vi "MagEncoder_cal_v1.vi"() -> ()   [LabVIEW 2014]
uses:
  <vilib>/eio/EIONode/EIONode.xnode
  <vilib>/rvi/eio/common/nirviEmuTemplateMethod_errors.vi
  <vilib>/rvi/Analysis/measure/butterworth/XNode/niFpgaButterworthFilter.xnode
  <vilib>/rvi/DataTransferAndStorage/Container/XNode/niFpgaContainer.xnode
  <vilib>/rvi/FXPMathLib/FxpSinAndCos/XNode/nifxpmath_SinAndCos.xnode
  <vilib>/rvi/FXPMathLib/FxpSinAndCos/simVIs/DllFxpSinAndCosTemp_sub.vi
  <vilib>/rvi/FXPMathLib/FxpSinAndCos/subVIs/nifxpmath_SinAndCos_SimConfig.ctl
  <vilib>/rvi/interface/RandomDataEmulation/nirviRandomDataFpgaMultiElementTemplate.vi
panel:
  in  "Vy (mm/s)":fxp<+/-,30,6>
  out "Dyr_ramp":fxp<+/-,22,7>
  in  "Dyr_stroke":fxp<+/-,32,7>
  out "Dpr_ramp":fxp<+/-,22,7>
  in  "Dpr_stroke":fxp<+/-,32,7>
  in  "Vp (mm/s)":fxp<+/-,30,6>
  out "omega_p (Mavg w. f)":fxp<+/-,36,18>
  in  "scaled coefficients":i32[](array[numeric])=[946630756, 63555534]
  in  "FIFO":i16(ring) items=["Pitch_F+P", "imp ctrl", "Yaw_F+P"]
  out "PID (kHz)":fxp<+/-,20,10>
  in  "Set 6":bool
  in  "Set 5":bool
  in  "Set 4":bool
  in  "Set 3":bool
  in  "Set 2":bool
  in  "Set 1":bool
  out "Dy1_d (T)":fxp<+/-,36,13>
  out "omega_y1 (T)":fxp<+/-,36,13>
  out "Dp1_d (T)":fxp<+/-,36,13>
  out "omega_p1 (T)":fxp<+/-,36,13>
  out "Dy2_d (T)":fxp<+/-,36,13>
  out "Dp2_d (T)":fxp<+/-,36,13>
  out "omega_y2 (T)":fxp<+/-,36,13>
  out "omega_p2 (T)":fxp<+/-,36,13>
  out "mt_omega_y2":u32
  out "mt_omega_p2":u32
  out "rad_y2":fxp<+/-,33,20>
  out "D_y2":fxp<+/-,32,7>
  out "rad_y1":fxp<+/-,33,20>
  out "D_y1":fxp<+/-,32,7>
  out "Encoder Position_y1":i32
  out "Encoder Position_y2":i32
  out "Encoder Position_p2":i32
  out "D_p2":fxp<+/-,32,7>
  out "rad_p2":fxp<+/-,33,20>
  out "D_p1":fxp<+/-,32,7>
  out "rad_p1":fxp<+/-,33,20>
  out "Encoder Position_p1":i32
  in  "Mag. factor_y":fxp<+/-,20,3>
  in  "Mag. encoder_y":bool
  out "omega_y (rad/s)":fxp<+/-,36,13>
  out "Dy_d (mm/s)":fxp<+/-,36,13>
  in  "Vy. Est.":i16(ring) items=["T", "Mavg"]
  out "omega_y (Mavg)":fxp<+/-,36,14>
  out "Dy_d (Mavg)":fxp<+/-,36,14>
  in  "Dy_d_M_avg_Tc (uSec)":i32
  out "Dp_d (Mavg)":fxp<+/-,36,14>
  out "omega_p (Mavg)":fxp<+/-,36,14>
  in  "Dp_d_M_avg_Tc (uSec)":i32
  out "Dp_d (T)":fxp<+/-,36,13>
  out "omega_p (T)":fxp<+/-,36,13>
  in  "Vp. Est.":i16(ring) items=["T", "Mavg"]
  in  "Mag. factor_p":fxp<+/-,20,3>
  in  "Mag. encoder_p":bool
  in  "Belt_out_p":fxp<+/-,7,7>
  in  "Belt_in_p":fxp<+/-,6,6>
  in  "Belt_out_y":fxp<+/-,7,7>
  in  "Belt_in_y":fxp<+/-,6,6>
  in  "mt0_omega_p":u32
  in  "Encoder reset":bool
  out "Dpr_sin":fxp<+/-,22,7>
  in  "Sin offset_p":fxp<+/-,22,7>
  in  "Sin magnitude_p":fxp<+/-,21,6>
  out "Dpr_sin_dd":fxp<+/-,35,20>
  out "Dpr_sin_d":fxp<+/-,33,15>
  out "Sin omega_p":fxp<+/-,34,9>
  in  "Sin wave freq._p (Hz)":fxp<+/-,32,6>
  in  "Dpr_step":fxp<+/-,22,7>
  out "Dpr_for":fxp<+/-,22,7>
  in  "Command_p":i16(ring) items=["Step", "Sine", "Ramp"]
  out "Fp_PID":fxp<+/-,36,16>
  in  "Kp_p":fxp<+/-,32,13>
  out "va_p":fxp<+/-,36,7>
  out "vb_p":fxp<+/-,37,8>
  out "vq_p_F":fxp<+/-,20,5> format="%.57g"
  out "vd_p_F":fxp<+/-,20,5>
  in  "Stop motor_p":bool
  out "Dp_d (mm/s)":fxp<+/-,36,13>
  out "omega_p (rad/s)":fxp<+/-,36,13>
  out "mt_omega_p1":u32
  out "rad_p(NrTheta)":fxp<+/-,33,20>
  out "D_p(mm)":fxp<+/-,32,7>
  out "Encoder Position_p":i32
  in  "Encoder reset_p":bool
  out "Dyr_for":fxp<+/-,22,7>
  in  "Command_y":i16(ring) items=["Step", "Sine", "Ramp"]
  out "vb_y":fxp<+/-,38,8>
  out "va_y":fxp<+/-,38,8>
  out "Dyr_sin_dd":fxp<+/-,35,20>
  out "Dyr_sin_d":fxp<+/-,33,15>
  out "Sin omega_y":fxp<+/-,34,9>
  out "Dyr_sin":fxp<+/-,22,7>
  in  "Sin offset_y":fxp<+/-,22,7>
  in  "Sin magnitude_y":fxp<+/-,21,6>
  out "Time now(s)":fxp<+,52,14>
  in  "Sin wave freq._y (Hz)":fxp<+/-,32,6>
  in  "Dyr_step":fxp<+/-,22,7>
  out "Fy_PID":fxp<+/-,36,16>
  in  "Kp_y":fxp<+/-,32,13>
  out "vq_y_F":fxp<+/-,20,5> format="%.57g"
  out "vd_y_F":fxp<+/-,20,5>
  in  "Stop motor_y":bool
  out "Dy_d (T)":fxp<+/-,36,13>
  out "omega_y (T)":fxp<+/-,36,13>
  in  "mt0_omega_y":u32
  out "mt_omega_y1":u32
  out "rad_y(NrTheta)":fxp<+/-,33,20>
  out "D_y(mm)":fxp<+/-,32,7>
  out "Encoder Position_y":i32
  in  "Encoder reset_y":bool
  in  "Ini coe.":bool
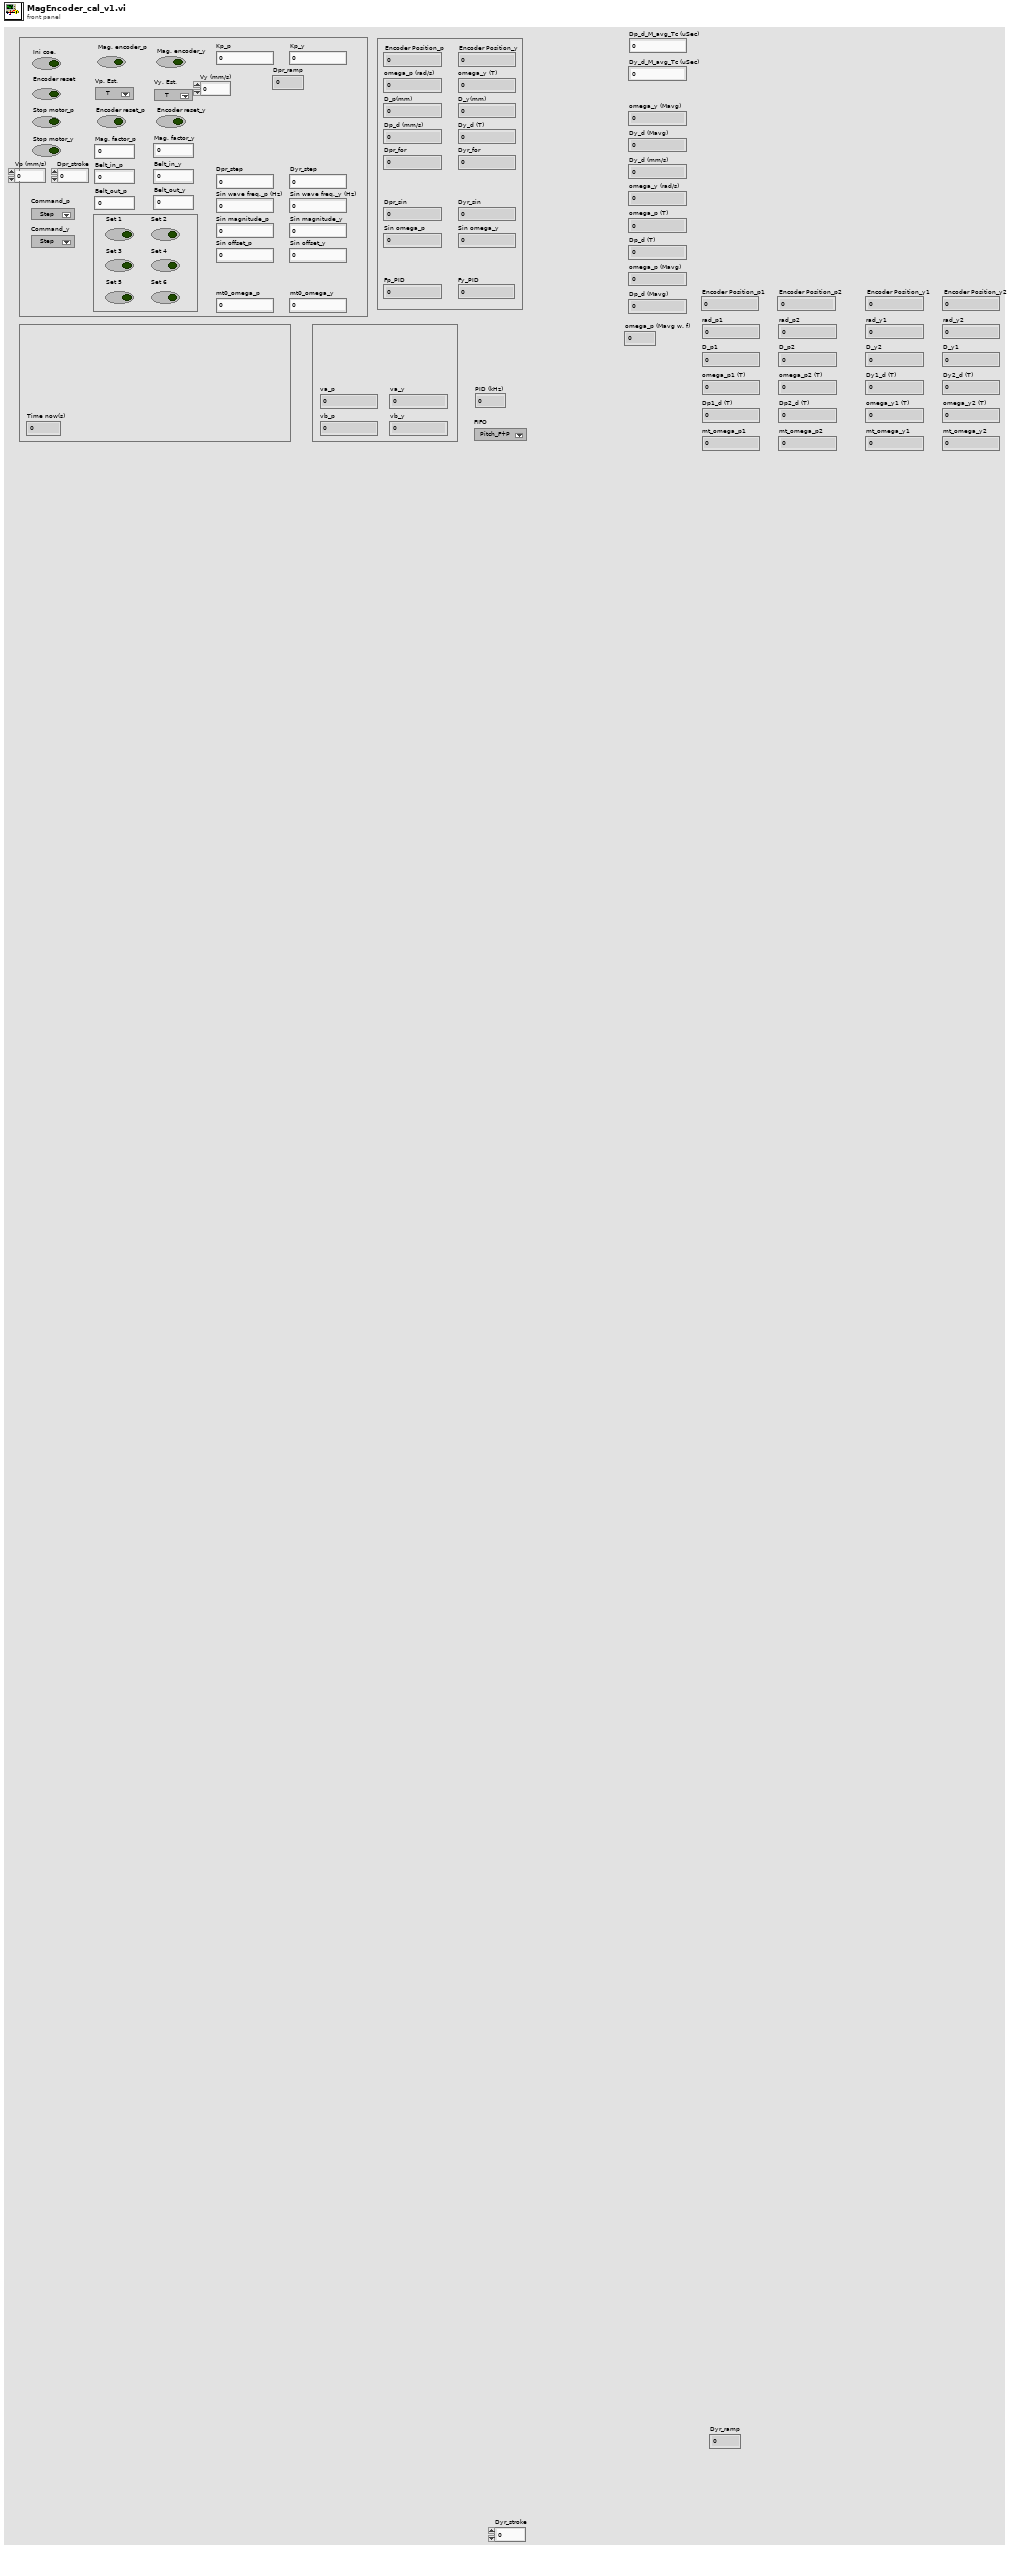
[diagram p1: front panel]
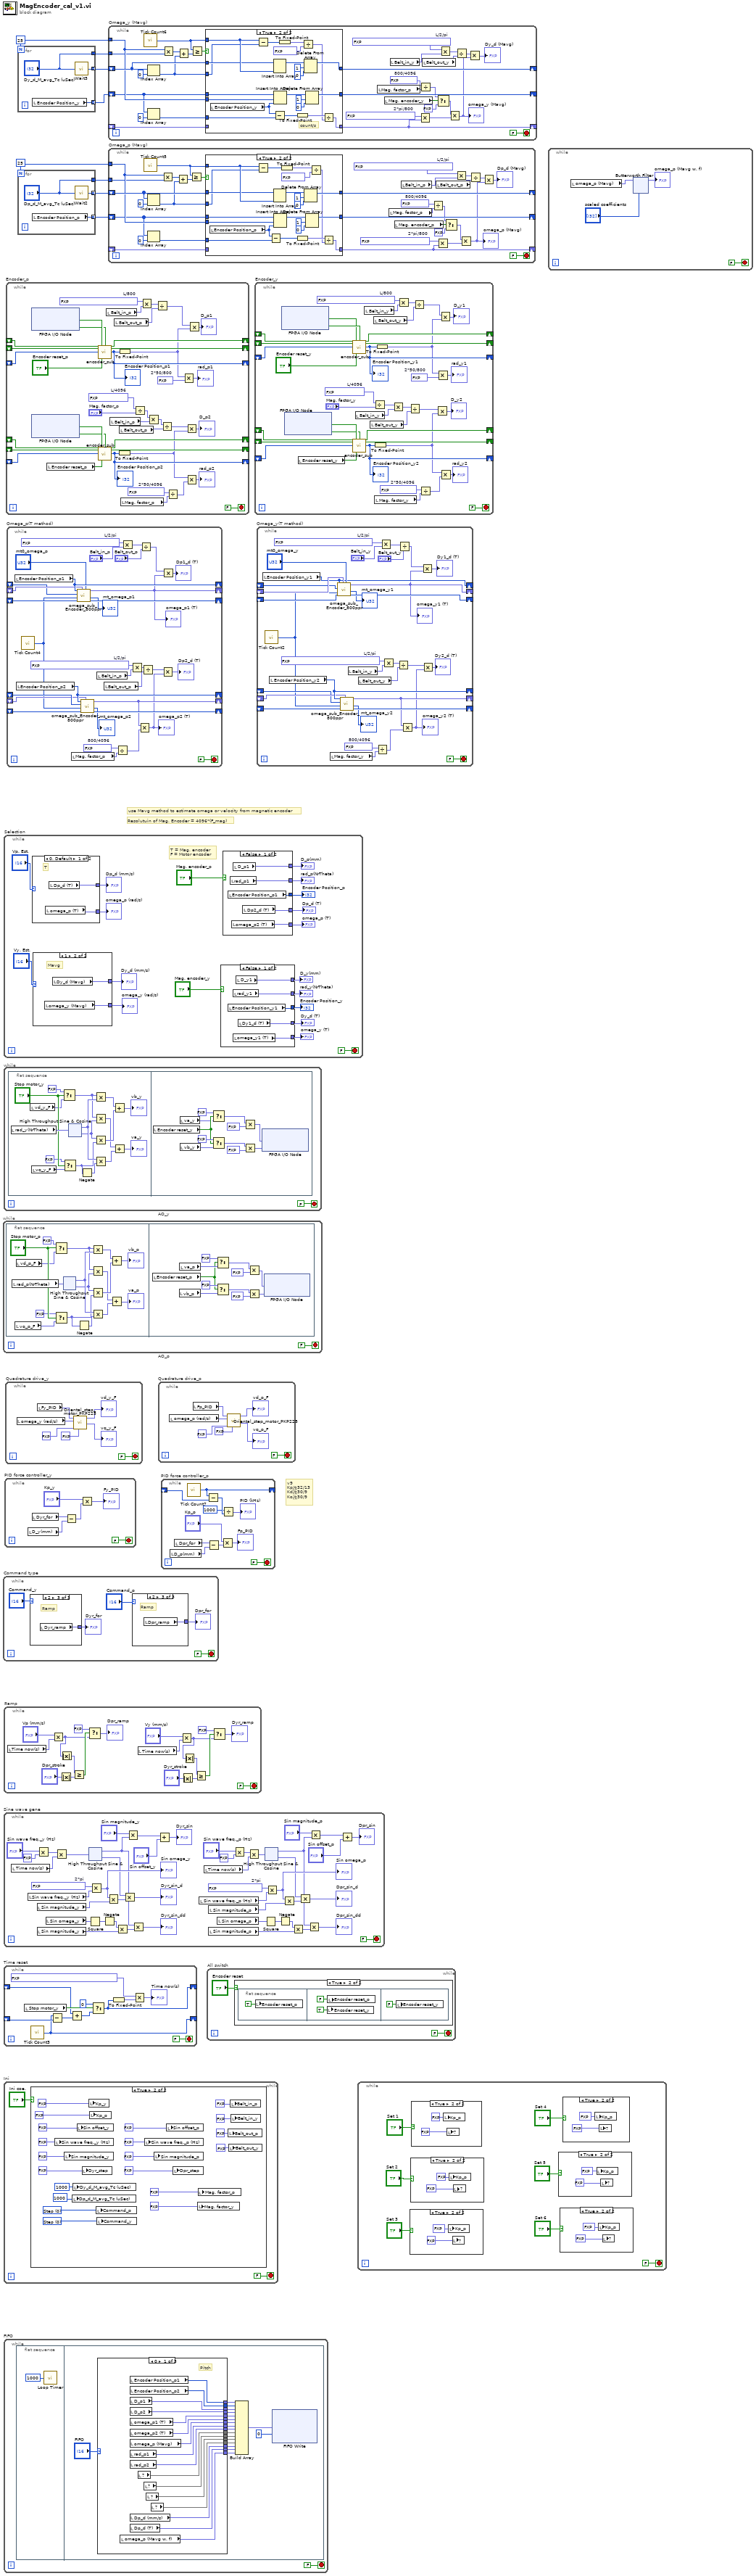
[diagram p0: block diagram]
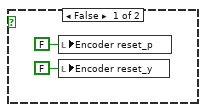
[diagram p10: hidden frame]
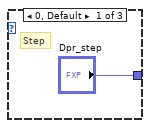
[diagram p11: hidden frame]
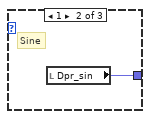
[diagram p12: hidden frame]
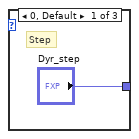
[diagram p13: hidden frame]
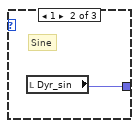
[diagram p14: hidden frame]
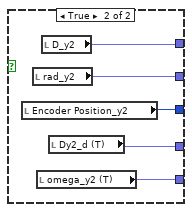
[diagram p15: hidden frame]
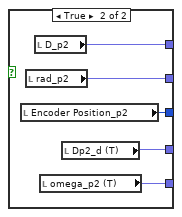
[diagram p16: hidden frame]
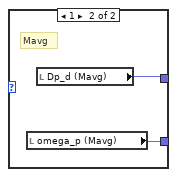
[diagram p17: hidden frame]
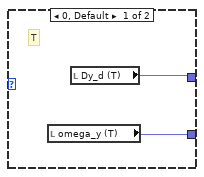
[diagram p18: hidden frame]
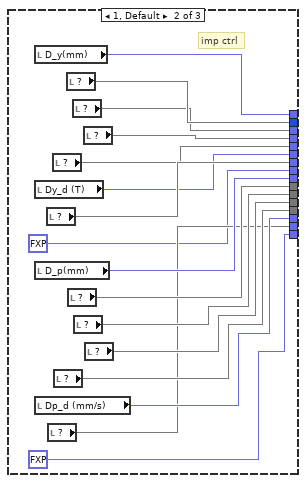
[diagram p20: hidden frame]
diagram:
  w5 = 25
  w8 = 25
  # "v9\nKp改32/13\nKd改30/9\nKo改30/9"
  # "Resolutuin of Mag. Encoder = 4096*(F_mag)"
  # "use Mavg method to estimate omega or velocity from magnetic encoder"
  n1 = while "AO_p" {
    stop <- FALSE stop-if-true
    n2 = flat-sequence {
      frame #0 {
        n3 = local read "rad_p(NrTheta)"() -> (w21:fxp<+/-,33,20>)
        n4 = local read "vq_p_F"() -> (w22:fxp<+/-,20,5>)
        n5 = local read "vd_p_F"() -> (w24:fxp<+/-,20,5>)
        n6 = Select(t=fxp<+/-,20,5> 0.0, s="Stop motor_p", f=w24) -> (s? t:f=w13:fxp<+/-,20,5>)
        n7 = Select(t=fxp<+,1,1> 0.0, s="Stop motor_p", f=w22) -> (s? t:f=w12:fxp<+/-,20,5>)
        n8 = xnode "High Throughput Sine & Cosine"("x (pi)"=w21) -> ("sin(x)"=w15:fxp<+/-,16,2>, "cos(x)"=w14:fxp<+/-,16,2>)
        n9 = Negate(x=w12) -> (-x=w20:fxp<+/-,21,6>)
        n10 = Multiply(x=w13, y=w15) -> (x*y=w19:fxp<+/-,36,7>)
        n11 = Multiply(x=w13, y=w14) -> (x*y=w17:fxp<+/-,36,7>)
        n12 = Multiply(x=w14, y=w12) -> (x*y=w18:fxp<+/-,36,7>)
        n13 = Multiply(x=w15, y=w20) -> (x*y=w16:fxp<+/-,35,6>)
        n14 = Add(x=w19, y=w18) -> (x+y=→"vb_p":fxp<+/-,37,8>)
        n15 = Add(x=w17, y=w16) -> (x+y=→"va_p":fxp<+/-,36,7>)
      }
      frame #1 {
        n16 = local read "Encoder reset_p"() -> (w57:bool)
        n17 = local read "vb_p"() -> (w58:fxp<+/-,37,8>)
        n18 = local read "va_p"() -> (w59:fxp<+/-,36,7>)
        n19 = Select(t=fxp<+,2,2> 3.0, s=w57, f=w59) -> (s? t:f=w65:fxp<+/-,36,7>)
        n20 = Select(t=fxp<+,1,1> 0.0, s=w57, f=w58) -> (s? t:f=w64:fxp<+/-,37,8>)
        n21 = Multiply(x=w65, y=fxp<+/-,1,0> -0.5) -> (x*y=w60:fxp<+/-,36,6>)
        n22 = Multiply(x=w64, y=fxp<+/-,1,0> -0.5) -> (x*y=w61:fxp<+/-,36,6>)
        n23 = xnode "FPGA I/O Node"("Mod8/AO0"=w60, "Mod8/AO1"=w61) -> ()  [unwired: 2 in, 2 out]
      }
    }
  }
  n24 = while "Command type" {
    stop <- FALSE stop-if-true
    n25 = case shown="2" "Command_y" {
      tunnel: ["Dyr_step" w77 w78] -> w71
      frame 0, Default {
        # "Step"
      }
      frame 1 {
        # "Sine"
        n26 = local read "Dyr_sin"() -> (w77:fxp<+/-,22,7>)
      }
      frame 2 {
        # "Ramp"
        n27 = local read "Dyr_ramp"() -> (w78:fxp<+/-,22,7>)
      }
    }
    "Dyr_for" <- w71
    n28 = case shown="2" "Command_p" {
      tunnel: ["Dpr_step" w74 w75] -> w69
      frame 0, Default {
        # "Step"
      }
      frame 1 {
        # "Sine"
        n29 = local read "Dpr_sin"() -> (w74:fxp<+/-,22,7>)
      }
      frame 2 {
        # "Ramp"
        n30 = local read "Dpr_ramp"() -> (w75:fxp<+/-,22,7>)
      }
    }
    "Dpr_for" <- w69
  }
  n31 = while "AO_y" {
    stop <- FALSE stop-if-true
    n32 = flat-sequence {
      frame #0 {
        n33 = local read "rad_y(NrTheta)"() -> (w96:fxp<+/-,33,20>)
        n34 = local read "vd_y_F"() -> (w94:fxp<+/-,20,5>)
        n35 = local read "vq_y_F"() -> (w93:fxp<+/-,20,5>)
        n36 = Select(t=fxp<+/-,20,5> 0.0, s="Stop motor_y", f=w94) -> (s? t:f=w88:fxp<+/-,20,5>)
        n37 = Select(t=fxp<+/-,20,5> 0.0, s="Stop motor_y", f=w93) -> (s? t:f=w87:fxp<+/-,20,5>)
        n38 = xnode "High Throughput Sine & Cosine"("x (pi)"=w96) -> ("sin(x)"=w90:fxp<+/-,17,2>, "cos(x)"=w89:fxp<+/-,17,2>)
        n39 = Negate(x=w87) -> (-x=w86:fxp<+/-,21,6>)
        n40 = Multiply(x=w88, y=w90) -> (x*y=w85:fxp<+/-,37,7>)
        n41 = Multiply(x=w88, y=w89) -> (x*y=w83:fxp<+/-,37,7>)
        n42 = Multiply(x=w89, y=w87) -> (x*y=w84:fxp<+/-,37,7>)
        n43 = Multiply(x=w90, y=w86) -> (x*y=w82:fxp<+/-,36,6>)
        n44 = Add(x=w85, y=w84) -> (x+y=→"vb_y":fxp<+/-,38,8>)
        n45 = Add(x=w83, y=w82) -> (x+y=→"va_y":fxp<+/-,37,7>)
      }
      frame #1 {
        n46 = local read "Encoder reset_y"() -> (w129:bool)
        n47 = local read "va_y"() -> (w128:fxp<+/-,38,8>)
        n48 = local read "vb_y"() -> (w127:fxp<+/-,38,8>)
        n49 = Select(t=fxp<+,2,2> 3.0, s=w129, f=w128) -> (s? t:f=w133:fxp<+/-,38,8>)
        n50 = Select(t=fxp<+,1,1> 0.0, s=w129, f=w127) -> (s? t:f=w132:fxp<+/-,38,8>)
        n51 = Multiply(x=w133, y=fxp<+/-,1,0> -0.5) -> (x*y=w136:fxp<+/-,39,8>)
        n52 = Multiply(x=w132, y=fxp<+/-,1,0> -0.5) -> (x*y=w137:fxp<+/-,37,6>)
        n53 = xnode "FPGA I/O Node"("Mod8/AO2"=w136, "Mod8/AO3"=w137) -> ()  [unwired: 2 in, 2 out]
      }
    }
  }
  n54 = while "Sine wave gene" {
    stop <- FALSE stop-if-true
    w143 = fxp<+,20,3> 6.2831878662109375  # 2*pi
    w175 = fxp<+,20,3> 6.2831878662109375  # 2*pi
    n55 = local read "Time now(s)"() -> (w181:fxp<+,52,14>)
    n56 = local read "Sin wave freq._y (Hz)"() -> (w174:fxp<+/-,32,6>)
    n57 = Multiply(x="Sin wave freq._y (Hz)", y=fxp<+/-,10,3> 2.0) -> (x*y=w182:fxp<+/-,41,9>)
    n58 = local read "Sin magnitude_y"() -> (w172:fxp<+/-,21,6>)
    n59 = local read "Sin magnitude_y"() -> (w165:fxp<+/-,21,6>)
    n60 = local read "Sin omega_y"() -> (w168:fxp<+/-,34,9>)
    n61 = Multiply(x=w182, y=w181) -> (x*y=w180:fxp<+/-,41,19>)
    n62 = Square(x=w168) -> (x^2=w167:fxp<+,34,18>)
    n63 = xnode "High Throughput Sine & Cosine"("x (pi)"=w180) -> ("sin(x)"=w162:fxp<+/-,16,2>, "cos(x)"=w170:fxp<+/-,16,2>)
    n64 = Multiply(x=w175, y=w174) -> (x*y=w173:fxp<+/-,34,9>)
    "Sin omega_y" <- w173
    n65 = Negate(x=w167) -> (-x=w166:fxp<+/-,35,19>)
    n66 = Multiply(x=w173, y=w172) -> (x*y=w171:fxp<+/-,33,15>)
    n67 = Multiply(x=w166, y=w165) -> (x*y=w164:fxp<+/-,34,20>)
    n68 = Multiply(x=w170, y=w171) -> (x*y=→"Dyr_sin_d":fxp<+/-,33,15>)
    n69 = Multiply(x="Sin magnitude_y", y=w162) -> (x*y=w178:fxp<+/-,37,8>)
    n70 = Multiply(x=w162, y=w164) -> (x*y=→"Dyr_sin_dd":fxp<+/-,35,20>)
    n71 = Add(x=w178, y="Sin offset_y") -> (x+y=→"Dyr_sin":fxp<+/-,37,8>)
    n72 = local read "Sin wave freq._p (Hz)"() -> (w139:fxp<+/-,32,6>)
    n73 = local read "Time now(s)"() -> (w157:fxp<+,52,14>)
    n74 = local read "Sin magnitude_p"() -> (w140:fxp<+/-,21,6>)
    n75 = local read "Sin magnitude_p"() -> (w142:fxp<+/-,21,6>)
    n76 = local read "Sin omega_p"() -> (w141:fxp<+/-,34,9>)
    n77 = Multiply(x="Sin wave freq._p (Hz)", y=fxp<+/-,10,3> 2.0) -> (x*y=w161:fxp<+/-,42,9>)
    n78 = Multiply(x=w161, y=w157) -> (x*y=w158:fxp<+/-,41,19>)
    n79 = Square(x=w141) -> (x^2=w153:fxp<+,34,18>)
    n80 = xnode "High Throughput Sine & Cosine"("x (pi)"=w158) -> ("sin(x)"=w144:fxp<+/-,16,2>, "cos(x)"=w149:fxp<+/-,16,2>)
    n81 = Multiply(x=w143, y=w139) -> (x*y=w156:fxp<+/-,34,9>)
    "Sin omega_p" <- w156
    n82 = Negate(x=w153) -> (-x=w152:fxp<+/-,35,19>)
    n83 = Multiply(x=w156, y=w140) -> (x*y=w155:fxp<+/-,33,15>)
    n84 = Multiply(x=w152, y=w142) -> (x*y=w151:fxp<+/-,35,19>)
    n85 = Multiply(x=w149, y=w155) -> (x*y=→"Dpr_sin_d":fxp<+/-,33,15>)
    n86 = Multiply(x=w144, y=w151) -> (x*y=→"Dpr_sin_dd":fxp<+/-,35,20>)
    n87 = Multiply(x="Sin magnitude_p", y=w144) -> (x*y=w147:fxp<+/-,37,8>)
    n88 = Add(x=w147, y="Sin offset_p") -> (x+y=→"Dpr_sin":fxp<+/-,37,8>)
  }
  n89 = while "Time reset" {
    shift-right: [w254] -> _
    shift-left: _ -> [w255]
    shift-right: [w249] -> _
    shift-left: _ -> [w250]
    stop <- FALSE stop-if-true
    n90 = local read "Stop motor_y"() -> (w256:bool)
    n91 = call "Tick Count3"() -> ("Tick Count(uSec)"=w254:u32)
    n92 = Subtract(x=w254, y=w255) -> (x-y=w253:u32)
    n93 = Add(x=w250, y=w253) -> (x+y=w252:u32)
    n94 = Select(t=u32 0, s=w256, f=w252) -> (s? t:f=w249:u32)
    n95 = To Fixed-Point(number=w249) -> (fixed-point=w248:fxp<+,32,32>)  [unwired: 1 in]
    n96 = Multiply(x=fxp<+,20,-18> 1.0000003385357559e-06, y=w248) -> (x*y=→"Time now(s)":fxp<+,52,14>)
  }
  n97 = while "Ini" {
    stop <- FALSE stop-if-true
    n98 = case shown="True" "Ini coe." {
      frame False {
      }
      frame True {
        w272 = i16 0 items=["Step", "Sine"] ("Command_p")
        w273 = i16 0 items=["Step", "Sine"] ("Command_y")
        n99 = local write "Sin wave freq._y (Hz)"(fxp<+/-,32,6> 1.0 ("Sin wave freq. (Hz)")) -> ()
        n100 = local write "Sin magnitude_y"(fxp<+/-,22,7> 5.0 ("Sin magnitude")) -> ()
        n101 = local write "Dp_d_M_avg_Tc (uSec)"(u32 1000 ("D_d_M_avg_Tc (uSec)")) -> ()
        n102 = local write "Dy_d_M_avg_Tc (uSec)"(1000 ("Dy_d_M_avg_Tc (uSec)")) -> ()
        n103 = local write "Sin offset_y"(fxp<+/-,38,9> 0.0 ("Sin offset")) -> ()
        n104 = local write "Dyr_step"(fxp<+/-,22,7> 0.0 ("Dr")) -> ()
        n105 = local write "Kp_y"(fxp<+/-,36,9> 30.0 ("Kp")) -> ()
        n106 = local write "Kp_p"(fxp<+/-,36,9> 30.0 ("Kp_p")) -> ()
        n107 = local write "Command_p"(w272) -> ()
        n108 = local write "Command_y"(w273) -> ()
        n109 = local write "Sin wave freq._p (Hz)"(fxp<+/-,32,6> 1.0 ("Sin wave freq._p (Hz)")) -> ()
        n110 = local write "Sin magnitude_p"(fxp<+/-,21,6> 5.0 ("Sin magnitude_p")) -> ()
        n111 = local write "Sin offset_p"(fxp<+/-,22,7> 0.0 ("Sin offset_p")) -> ()
        n112 = local write "Dpr_step"(fxp<+/-,22,7> 0.0 ("Dpr_step")) -> ()
        n113 = local write "Mag. factor_y"(fxp<+/-,36,9> 1.0 ("Kd_p")) -> ()
        n114 = local write "Mag. factor_p"(fxp<+/-,36,9> 1.0 ("Ki_p")) -> ()
        n115 = local write "Belt_out_p"(fxp<+/-,7,7> 22.0 ("Belt_op")) -> ()
        n116 = local write "Belt_out_y"(fxp<+/-,7,7> 22.0 ("Belt_oy")) -> ()
        n117 = local write "Belt_in_p"(fxp<+/-,6,6> 16.0 ("Belt_mp")) -> ()
        n118 = local write "Belt_in_y"(fxp<+/-,6,6> 16.0 ("Belt_my")) -> ()
      }
    }
  }
  n119 = while "FIFO" {
    stop <- FALSE stop-if-true
    n120 = flat-sequence {
      frame #0 {
        n121 = call "Loop Timer"("Count(uSec)"=u32 1000) -> ()  [unwired: 1 out]
      }
      frame #1 {
        n122 = case shown="0" "FIFO" {
          tunnel: [w315 w331 w347] -> w299
          tunnel: [w314 w330 w346] -> w298
          tunnel: [w313 w329 w345] -> w297
          tunnel: [w312 w328 w344] -> w296
          tunnel: [w309 w327 w341] -> w294
          tunnel: [w310 w326 w342] -> w293
          tunnel: [w311 w325 w343] -> w292
          tunnel: [w307 w324 w339] -> w291
          tunnel: [w306 w323 w338] -> w290
          tunnel: [w305 w322 w337] -> w289
          tunnel: [w304 w321 w336] -> w288
          tunnel: [w303 w320 w335] -> w287
          tunnel: [w302 w319 w334] -> w286
          tunnel: [w301 w318 w333] -> w285
          tunnel: [w300 fxp<+,1,1> 0.0 ("element") w332] -> w284
          tunnel: [w308 fxp<+,1,1> 0.0 w340] -> w282
          frame 0 {
            # "Pitch"
            n123 = local read "omega_p (Mavg w. f)"() -> (w300:fxp<+/-,36,18>)
            n124 = local read "Encoder Position_p1"() -> (w315:i32)
            n125 = local read "Encoder Position_p2"() -> (w314:i32)
            n126 = local read "D_p1"() -> (w313:fxp<+/-,32,7>)
            n127 = local read "D_p2"() -> (w312:fxp<+/-,32,7>)
            n128 = local read "omega_p1 (T)"() -> (w311:fxp<+/-,36,13>)
            n129 = local read "omega_p2 (T)"() -> (w310:fxp<+/-,36,13>)
            n130 = local read "omega_p (Mavg)"() -> (w309:fxp<+/-,36,14>)
            n131 = local read "rad_p1"() -> (w308:fxp<+/-,33,20>)
            n132 = local read "rad_p2"() -> (w307:fxp<+/-,33,20>)
            n133 = local read "Dp_d (mm/s)"() -> (w302:fxp<+/-,36,13>)
            n134 = local read "Dp_d (T)"() -> (w301:fxp<+/-,36,13>)
            n135 = local read item#-1() -> (w306)
            n136 = local read item#-1() -> (w305)
            n137 = local read item#-1() -> (w304)
            n138 = local read item#-1() -> (w303)
          }
          frame 1, Default {
            # "imp ctrl"
            n139 = local read "D_y(mm)"() -> (w331:fxp<+/-,32,7>)
            n140 = local read "Dy_d (T)"() -> (w326:fxp<+/-,36,13>)
            n141 = local read "D_p(mm)"() -> (w324:fxp<+/-,32,7>)
            n142 = local read "Dp_d (mm/s)"() -> (w319:fxp<+/-,36,13>)
            n143 = local read item#-1() -> (w327)
            n144 = local read item#-1() -> (w318)
            n145 = local read item#-1() -> (w325)
            n146 = local read item#-1() -> (w320)
            n147 = local read item#-1() -> (w330)
            n148 = local read item#-1() -> (w323)
            n149 = local read item#-1() -> (w329)
            n150 = local read item#-1() -> (w322)
            n151 = local read item#-1() -> (w328)
            n152 = local read item#-1() -> (w321)
          }
          frame 2 {
            # "Yaw"
            n153 = local read "Encoder Position_y1"() -> (w347:i32)
            n154 = local read "Encoder Position_y2"() -> (w346:i32)
            n155 = local read "D_y1"() -> (w345:fxp<+/-,32,7>)
            n156 = local read "D_y2"() -> (w344:fxp<+/-,32,7>)
            n157 = local read "omega_y1 (T)"() -> (w343:fxp<+/-,36,13>)
            n158 = local read "omega_y2 (T)"() -> (w342:fxp<+/-,36,13>)
            n159 = local read "omega_y (Mavg)"() -> (w341:fxp<+/-,36,14>)
            n160 = local read "rad_y1"() -> (w340:fxp<+/-,33,20>)
            n161 = local read "rad_y2"() -> (w339:fxp<+/-,33,20>)
            n162 = local read "Dy_d (mm/s)"() -> (w334:fxp<+/-,36,13>)
            n163 = local read "Dy_d (T)"() -> (w333:fxp<+/-,36,13>)
            n164 = local read "Dy_d (Mavg)"() -> (w332:fxp<+/-,36,14>)
            n165 = local read item#-1() -> (w338)
            n166 = local read item#-1() -> (w337)
            n167 = local read item#-1() -> (w336)
            n168 = local read item#-1() -> (w335)
          }
        }
        n169 = Build Array(w299, w298, w297, w296, w292, w293, w294, w282, w291, w290, w289, w288, w287, w286, w285, w284) -> (w283:fxp<+/-,57,32>[])
        n170 = xnode ("FIFO Write")("Element"=w283, "Timeout"=0) -> ()  [unwired: 1 in, 2 out]
      }
    }
  }
  n171 = while "Selection" {
    stop <- FALSE stop-if-true
    # "T = Mag. encoder\nF = Motor encoder"
    n172 = case shown="0, Default" "Vp. Est." {
      tunnel: [w388 w389] -> w362
      tunnel: [w387 w390] -> w363
      frame 0, Default {
        # "T"
        n173 = local read "omega_p (T)"() -> (w388:fxp<+/-,36,13>)
        n174 = local read "Dp_d (T)"() -> (w387:fxp<+/-,36,13>)
      }
      frame 1 {
        # "Mavg"
        n175 = local read "omega_p (Mavg)"() -> (w389:fxp<+/-,36,14>)
        n176 = local read "Dp_d (Mavg)"() -> (w390:fxp<+/-,36,14>)
      }
    }
    "Dp_d (mm/s)" <- w363
    "omega_p (rad/s)" <- w362
    n177 = case shown="1" "Vy. Est." {
      tunnel: [w392 w394] -> w365
      tunnel: [w391 w393] -> w366
      frame 0, Default {
        # "T"
        n178 = local read "omega_y (T)"() -> (w391:fxp<+/-,36,13>)
        n179 = local read "Dy_d (T)"() -> (w392:fxp<+/-,36,13>)
      }
      frame 1 {
        # "Mavg"
        n180 = local read "omega_y (Mavg)"() -> (w393:fxp<+/-,36,14>)
        n181 = local read "Dy_d (Mavg)"() -> (w394:fxp<+/-,36,14>)
      }
    }
    "Dy_d (mm/s)" <- w365
    "omega_y (rad/s)" <- w366
    n182 = case shown="False" "Mag. encoder_y" {
      tunnel: [w371 w375] -> w353
      tunnel: [w370 w376] -> w354
      tunnel: [w369 w374] -> w356
      tunnel: [w367 w373] -> w350
      tunnel: [w368 w372] -> w349
      frame False {
        n183 = local read "Encoder Position_y1"() -> (w369:i32)
        n184 = local read "rad_y1"() -> (w371:fxp<+/-,33,20>)
        n185 = local read "omega_y1 (T)"() -> (w367:fxp<+/-,36,13>)
        n186 = local read "D_y1"() -> (w370:fxp<+/-,32,7>)
        n187 = local read "Dy1_d (T)"() -> (w368:fxp<+/-,36,13>)
      }
      frame True {
        n188 = local read "Encoder Position_y2"() -> (w374:i32)
        n189 = local read "rad_y2"() -> (w375:fxp<+/-,33,20>)
        n190 = local read "omega_y2 (T)"() -> (w373:fxp<+/-,36,13>)
        n191 = local read "D_y2"() -> (w376:fxp<+/-,32,7>)
        n192 = local read "Dy2_d (T)"() -> (w372:fxp<+/-,36,13>)
      }
    }
    "D_y(mm)" <- w354
    "rad_y(NrTheta)" <- w353
    "Encoder Position_y" <- w356
    "Dy_d (T)" <- w349
    "omega_y (T)" <- w350
    n193 = case shown="False" "Mag. encoder_p" {
      tunnel: [w381 w386] -> w358
      tunnel: [w380 w385] -> w359
      tunnel: [w379 w384] -> w360
      tunnel: [w377 w383] -> w352
      tunnel: [w378 w382] -> w351
      frame False {
        n194 = local read "Encoder Position_p1"() -> (w379:i32)
        n195 = local read "rad_p1"() -> (w380:fxp<+/-,33,20>)
        n196 = local read "omega_p2 (T)"() -> (w377:fxp<+/-,36,13>)
        n197 = local read "D_p1"() -> (w381:fxp<+/-,32,7>)
        n198 = local read "Dp2_d (T)"() -> (w378:fxp<+/-,36,13>)
      }
      frame True {
        n199 = local read "Encoder Position_p2"() -> (w384:i32)
        n200 = local read "rad_p2"() -> (w385:fxp<+/-,33,20>)
        n201 = local read "D_p2"() -> (w386:fxp<+/-,32,7>)
        n202 = local read "omega_p2 (T)"() -> (w383:fxp<+/-,36,13>)
        n203 = local read "Dp2_d (T)"() -> (w382:fxp<+/-,36,13>)
      }
    }
    "D_p(mm)" <- w358
    "rad_p(NrTheta)" <- w359
    "Encoder Position_p" <- w360
    "Dp_d (T)" <- w351
    "omega_p (T)" <- w352
  }
  n204 = while "Ramp" {
    stop <- FALSE stop-if-true
    n205 = local read "Time now(s)"() -> (w412:fxp<+,52,14>)
    n206 = Multiply(x="Vp (mm/s)", y=w412) -> (x*y=w399:fxp<+/-,64,20>)
    n207 = Absolute Value(x="Dpr_stroke") -> (abs(x)=w401:fxp<+,32,7>)
    n208 = Absolute Value(x=w399) -> (abs(x)=w400:fxp<+,64,20>)
    n209 = Greater Or Equal?(x=w400, y=w401) -> (x >= y?=w411:bool)
    n210 = Select(t=fxp<+/-,64,46> 0.0, s=w411, f=w399) -> (s? t:f=→"Dpr_ramp":fxp<+/-,64,46>)
    n211 = local read "Time now(s)"() -> (w405:fxp<+,52,14>)
    n212 = Multiply(x="Vy (mm/s)", y=w405) -> (x*y=w395:fxp<+/-,64,20>)
    n213 = Absolute Value(x="Dyr_stroke") -> (abs(x)=w397:fxp<+,32,7>)
    n214 = Absolute Value(x=w395) -> (abs(x)=w396:fxp<+,64,20>)
    n215 = Greater Or Equal?(x=w396, y=w397) -> (x >= y?=w408:bool)
    n216 = Select(t=fxp<+/-,64,46> 0.0, s=w408, f=w395) -> (s? t:f=→"Dyr_ramp":fxp<+/-,64,46>)
  }
  n217 = while "PID force controller_y" {
    stop <- FALSE stop-if-true
    n218 = local read "D_y(mm)"() -> (w417:fxp<+/-,32,7>)
    n219 = local read "Dyr_for"() -> (w418:fxp<+/-,22,7>)
    n220 = Subtract(x=w418, y=w417) -> (x-y=w416:fxp<+/-,33,8>)
    n221 = Multiply(x="Kp_y", y=w416) -> (x*y=→"Fy_PID":fxp<+/-,64,20>)
  }
  n222 = while "Quadrature drive_y" {
    stop <- FALSE stop-if-true
    n223 = local read "omega_y (rad/s)"() -> (w426:fxp<+/-,36,13>)
    n224 = local read "Fy_PID"() -> (w422:fxp<+/-,36,16>)
    n225 = call "Oriental_step_motor_PKP225.vi"("F_Threshold"=fxp<+,12,12> 10.0, "dFmr"=fxp<+/-,25,15> 0.0, "omega"=w426, "Fmr"=w422) -> ("vq_F"=→"vq_y_F":fxp<+/-,20,5>, "vd_F"=→"vd_y_F":fxp<+/-,20,5>)  [unwired: 6 in]
  }
  n226 = while "Encoder_p" {
    shift-right: [w464] -> _
    shift-left: _ -> [w463]
    shift-right: [w465] -> _
    shift-left: _ -> [w462]
    shift-right: [w459] -> _
    shift-left: _ -> [w461]
    shift-right: [w450] -> _
    shift-left: _ -> [w449]
    shift-right: [w451] -> _
    shift-left: _ -> [w452]
    shift-right: [w446] -> _
    shift-left: _ -> [w447]
    stop <- FALSE stop-if-true
    w442 = fxp<+/-,20,-5> 0.00048828125  # L/4096
    w440 = fxp<+/-,16,1> 0.0244140625  # 2*50/4096
    w458 = fxp<+/-,20,-5> 0.002499997615814209  # L/800
    w432 = fxp<+/-,16,1> 0.125  # 2*50/800
    n227 = xnode "FPGA I/O Node"() -> ("Mod7/DIO0"=w467:bool, "Mod7/DIO1"=w466:bool)  [unwired: 2 in, 2 out]
    n228 = xnode "FPGA I/O Node"() -> ("Mod7/DIO4"=w454:bool, "Mod7/DIO5"=w453:bool)  [unwired: 2 in, 2 out]
    n229 = local read "Encoder reset_p"() -> (w448:bool)
    n230 = call "encoder_sub.vi"("A_pre"=w463, "B_pre"=w462, "Encoder Position_pre"=w461, "A input"=w467, "Encoder Position Reset"="Encoder reset_p", "B input"=w466) -> ("A"=w464:bool, "B"=w465:bool, "Encoder Position (Counts)"=w459:i32)  [unwired: 19 in]
    "Encoder Position_p1" <- w459
    n231 = call "encoder_sub.vi"("A_pre"=w449, "B_pre"=w452, "Encoder Position_pre"=w447, "A input"=w454, "Encoder Position Reset"=w448, "B input"=w453) -> ("A"=w450:bool, "B"=w451:bool, "Encoder Position (Counts)"=w446:i32)  [unwired: 19 in]
    "Encoder Position_p2" <- w446
    n232 = local read "Belt_in_p"() -> (w457:fxp<+/-,6,6>)
    n233 = local read "Belt_in_p"() -> (w443:fxp<+/-,6,6>)
    n234 = local read "Belt_out_p"() -> (w455:fxp<+/-,7,7>)
    n235 = To Fixed-Point(number=w446) -> (fixed-point=w428:fxp<+/-,32,32>)  [unwired: 1 in]
    n236 = To Fixed-Point(number=w459) -> (fixed-point=w433:fxp<+/-,32,32>)  [unwired: 1 in]
    n237 = local read "Belt_out_p"() -> (w445:fxp<+/-,7,7>)
    n238 = local read "Mag. factor_p"() -> (w439:fxp<+/-,20,3>)
    n239 = Divide(x=w442, y="Mag. factor_p") -> (x/y=w441:fxp<+/-,41,13>)
    n240 = Multiply(x=w458, y=w457) -> (x*y=w456:fxp<+/-,26,1>)
    n241 = Multiply(x=w441, y=w443) -> (x*y=w444:fxp<+/-,46,18>)
    n242 = Divide(x=w456, y=w455) -> (x/y=w435:fxp<+/-,33,1>)
    n243 = Divide(x=w444, y=w445) -> (x/y=w430:fxp<+/-,53,18>)
    n244 = Divide(x=w440, y=w439) -> (x/y=w427:fxp<+/-,32,1>)
    n245 = Multiply(x=w433, y=w432) -> (x*y=→"rad_p1":fxp<+/-,33,20>)
    n246 = Multiply(x=w430, y=w428) -> (x*y=→"D_p2":fxp<+/-,37,7>)
    n247 = Multiply(x=w428, y=w427) -> (x*y=→"rad_p2":fxp<+/-,33,20>)
    n248 = Multiply(x=w435, y=w433) -> (x*y=→"D_p1":fxp<+/-,32,7>)
  }
  n249 = while "Omega_p(T method)" {
    shift-right: [w500] -> _
    shift-left: _ -> [w498]
    shift-right: [w471] -> _
    shift-left: _ -> [w499]
    shift-right: [w496] -> _
    shift-left: _ -> [w497]
    shift-right: [w487] -> _
    shift-left: _ -> [w486]
    shift-right: [w480] -> _
    shift-left: _ -> [w485]
    shift-right: [w484] -> _
    shift-left: _ -> [w483]
    stop <- FALSE stop-if-true
    w478 = fxp<+/-,32,0> 0.3183098859153688  # L/2/pi
    w489 = fxp<+,32,0> 0.1953125  # 800/4096
    w493 = fxp<+/-,32,0> 0.3183098859153688  # L/2/pi
    n250 = local read "Encoder Position_p1"() -> (w500:i32)
    n251 = local read "Encoder Position_p2"() -> (w487:i32)
    n252 = call "Tick Count4"() -> ("Tick Count(Ticks)"=w482:u32)
    n253 = local read "Mag. factor_p"() -> (w488:fxp<+/-,20,3>)
    n254 = call "omega_sub_Encoder_800ppr.vi"("mt0"="mt0_omega_p", "omega_pre"=w499, "ticks_m_pre"=w497, "ticks"=w482, "count_pre"=w498, "count"=w500) -> ("ticks_m"=w496:u32, "mt"=→"mt_omega_p1":u32, "omega"=w471:fxp<+/-,36,13>)  [unwired: 3 in]
    "omega_p1 (T)" <- w471
    n255 = call "omega_sub_Encoder_800ppr.vi"("omega_pre"=w485, "ticks_m_pre"=w483, "ticks"=w482, "count_pre"=w486, "count"=w487) -> ("ticks_m"=w484:u32, "mt"=→"mt_omega_p2":u32, "omega"=w480:fxp<+/-,36,13>)  [unwired: 4 in]
    n256 = local read "Belt_in_p"() -> (w476:fxp<+/-,6,6>)
    n257 = local read "Belt_out_p"() -> (w475:fxp<+/-,7,7>)
    n258 = Divide(x=w489, y=w488) -> (x/y=w479:fxp<+/-,32,1>)
    n259 = Multiply(x=w493, y="Belt_in_p") -> (x*y=w491:fxp<+/-,38,6>)
    n260 = Multiply(x=w478, y=w476) -> (x*y=w477:fxp<+/-,38,6>)
    n261 = Multiply(x=w480, y=w479) -> (x*y=w469:fxp<+/-,36,13>)
    "omega_p2 (T)" <- w469
    n262 = Divide(x=w491, y="Belt_out_p") -> (x/y=w472:fxp<+/-,20,1>)
    n263 = Divide(x=w477, y=w475) -> (x/y=w470:fxp<+/-,45,6>)
    n264 = Multiply(x=w470, y=w469) -> (x*y=→"Dp2_d (T)":fxp<+/-,36,13>)
    n265 = Multiply(x=w472, y=w471) -> (x*y=→"Dp1_d (T)":fxp<+/-,36,13>)
  }
  n266 = for {
    N: w5 -> [_]
    tunnel: [w503] -> w4 mode=indexing
    tunnel: [w502] -> w3 mode=indexing
    tunnel: ["Dy_d_M_avg_Tc (uSec)"] -> w2
    n267 = local read "Encoder Position_y"() -> (w502:i32)
    n268 = call "Wait3"("Count(uSec)"="Dy_d_M_avg_Tc (uSec)") -> ("Tick Count(uSec)"=w503:u32)
  }
  n269 = for {
    N: w8 -> [_]
    tunnel: ["Dp_d_M_avg_Tc (uSec)"] -> w1
    tunnel: [w505] -> w7 mode=indexing
    tunnel: [w504] -> w6 mode=indexing
    n270 = local read "Encoder Position_p"() -> (w504:i32)
    n271 = call "Wait2"("Count(uSec)"="Dp_d_M_avg_Tc (uSec)") -> ("Tick Count(uSec)"=w505:u32)
  }
  n272 = while "Omega_y (Mavg)" {
    tunnel: w5 -> [w530]
    shift-right: [w528] -> _
    shift-left: w4 -> [w533]
    shift-right: [w527] -> _
    shift-left: w3 -> [w529]
    shift-right: [w522] -> _
    shift-left: _ -> [w526]
    tunnel: w2 -> [w521]
    stop <- FALSE stop-if-true
    w509 = fxp<+/-,32,0> 0.3183098859153688  # L/2/pi
    w518 = fxp<+,32,0> 0.1953125  # 800/4096
    w524 = fxp<+/-,27,3> 0.007853984832763672  # 2*pi/800
    n273 = call "Tick Count6"() -> ("Tick Count(uSec)"=w534:u32)
    n274 = Index Array(array=w533, index=0) -> (element=w532:u32)
    n275 = Index Array(array=w529, index=0) -> (element=w531:i32)
    n276 = Multiply(x=w530, y=w521) -> (x*y=w536:i32)
    n277 = Add(x=w536, y=w532) -> (x+y=w535:u32)
    n278 = Greater Or Equal?(x=w534, y=w535) -> (x >= y?=w525:bool)
    n279 = case shown="True" w525 {
      tunnel: w534 -> [_ w557]
      tunnel: w530 -> [_ w554]
      tunnel: w533 -> [w541 w556]
      tunnel: w532 -> [_ w555]
      tunnel: w531 -> [_ w551]
      tunnel: w529 -> [w540 w553]
      tunnel: [w539 w549] -> w522
      tunnel: [w541 w548] -> w528
      tunnel: [w540 w547] -> w527
      tunnel: w526 -> [w539 _]
      frame False {
      }
      frame True {
        # "count/s"
        n280 = local read "Encoder Position_y"() -> (w550:i32)
        n281 = Subtract(x=w557, y=w555) -> (x-y=w558:u32)
        n282 = Insert Into Array(array=w556, new element=w557) -> (w560:u32[])  [unwired: 1 in]
        n283 = Subtract(x=w550, y=w551) -> (x-y=w545:i32)
        n284 = Insert Into Array(array=w553, index=w554, new element=w550) -> (w561:i32[])
        n285 = To Fixed-Point(number=w558) -> (fixed-point=w544:fxp<+,32,32>)  [unwired: 1 in]
        n286 = To Fixed-Point(number=w545) -> (fixed-point=w552:fxp<+/-,32,32>)  [unwired: 1 in]
        n287 = Divide(x=w544, y=fxp<+,32,32> 1000000.0) -> (x/y=w543:fxp<+/-,64,32>)
        n288 = Delete From Array(array=w560, length=1, index=0) -> (array with subset deleted=w548:u32[])  [unwired: 1 out]
        n289 = Delete From Array(array=w561, length=1, index=0) -> (array with subset deleted=w547:i32[])  [unwired: 1 out]
        n290 = Divide(x=w552, y=w543) -> (x/y=w549:fxp<+/-,40,20>)
      }
    }
    n291 = local read "Mag. factor_p"() -> (w517:fxp<+/-,20,3>)
    n292 = local read "Mag. encoder_y"() -> (w520:bool)
    n293 = local read "Belt_in_y"() -> (w511:fxp<+/-,6,6>)
    n294 = Multiply(x=w524, y=w522) -> (x*y=w514:fxp<+/-,44,14>)
    n295 = Divide(x=w518, y=w517) -> (x/y=w516:fxp<+/-,32,1>)
    n296 = local read "Belt_out_y"() -> (w512:fxp<+/-,7,7>)
    n297 = Select(t=w516, s=w520, f=fxp<+/-,2,2> 1.0) -> (s? t:f=w515:fxp<+/-,33,2>)
    n298 = Multiply(x=w509, y=w511) -> (x*y=w510:fxp<+/-,38,6>)
    n299 = Multiply(x=w515, y=w514) -> (x*y=w513:fxp<+/-,36,14>)
    "omega_y (Mavg)" <- w513
    n300 = Divide(x=w510, y=w512) -> (x/y=w508:fxp<+/-,45,6>)
    n301 = Multiply(x=w508, y=w513) -> (x*y=→"Dy_d (Mavg)":fxp<+/-,36,14>)
  }
  n302 = while "Omega_p (Mavg)" {
    tunnel: w8 -> [w587]
    shift-right: [w585] -> _
    shift-left: w7 -> [w590]
    shift-right: [w584] -> _
    shift-left: w6 -> [w586]
    shift-right: [w583] -> _
    shift-left: _ -> [w582]
    tunnel: w1 -> [w580]
    stop <- FALSE stop-if-true
    w569 = fxp<+/-,27,3> 0.007853984832763672  # 2*pi/800
    w571 = fxp<+,32,0> 0.1953125  # 800/4096
    w568 = fxp<+/-,32,0> 0.3183098859153688  # L/2/pi
    n303 = call "Tick Count5"() -> ("Tick Count(uSec)"=w591:u32)
    n304 = Index Array(array=w590, index=0) -> (element=w589:u32)
    n305 = Index Array(array=w586, index=0) -> (element=w588:i32)
    n306 = Multiply(x=w587, y=w580) -> (x*y=w593:i32)
    n307 = Add(x=w593, y=w589) -> (x+y=w592:u32)
    n308 = Greater Or Equal?(x=w591, y=w592) -> (x >= y?=w581:bool)
    n309 = case shown="True" w581 {
      tunnel: w591 -> [_ w614]
      tunnel: w587 -> [_ w611]
      tunnel: w590 -> [w598 w613]
      tunnel: w589 -> [_ w612]
      tunnel: w588 -> [_ w608]
      tunnel: w586 -> [w597 w610]
      tunnel: [w596 w606] -> w583
      tunnel: [w598 w605] -> w585
      tunnel: [w597 w604] -> w584
      tunnel: w582 -> [w596 _]
      frame False {
      }
      frame True {
        n310 = local read "Encoder Position_p"() -> (w607:i32)
        n311 = Subtract(x=w614, y=w612) -> (x-y=w615:u32)
        n312 = Subtract(x=w607, y=w608) -> (x-y=w599:i32)
        n313 = Insert Into Array(array=w613, new element=w614) -> (w617:u32[])  [unwired: 1 in]
        n314 = Insert Into Array(array=w610, index=w611, new element=w607) -> (w618:i32[])
        n315 = To Fixed-Point(number=w615) -> (fixed-point=w601:fxp<+,32,32>)  [unwired: 1 in]
        n316 = To Fixed-Point(number=w599) -> (fixed-point=w609:fxp<+/-,32,32>)  [unwired: 1 in]
        n317 = Delete From Array(array=w617, length=1, index=0) -> (array with subset deleted=w605:u32[])  [unwired: 1 out]
        n318 = Delete From Array(array=w618, length=1, index=0) -> (array with subset deleted=w604:i32[])  [unwired: 1 out]
        n319 = Divide(x=w601, y=fxp<+,32,32> 1000000.0) -> (x/y=w602:fxp<+/-,64,32>)
        n320 = Divide(x=w609, y=w602) -> (x/y=w606:fxp<+/-,40,20>)
      }
    }
    n321 = local read "Mag. factor_p"() -> (w572:fxp<+/-,20,3>)
    n322 = local read "Mag. encoder_p"() -> (w579:bool)
    n323 = local read "Belt_in_p"() -> (w576:fxp<+/-,6,6>)
    n324 = Divide(x=w571, y=w572) -> (x/y=w570:fxp<+/-,32,1>)
    n325 = local read "Belt_out_p"() -> (w575:fxp<+/-,7,7>)
    n326 = Multiply(x=w569, y=w583) -> (x*y=w577:fxp<+/-,44,14>)
    n327 = Select(t=w570, s=w579, f=fxp<+/-,2,2> 1.0) -> (s? t:f=w564:fxp<+/-,33,2>)
    n328 = Multiply(x=w568, y=w576) -> (x*y=w574:fxp<+/-,38,6>)
    n329 = Multiply(x=w564, y=w577) -> (x*y=w567:fxp<+/-,36,14>)
    "omega_p (Mavg)" <- w567
    n330 = Divide(x=w574, y=w575) -> (x/y=w566:fxp<+/-,45,6>)
    n331 = Multiply(x=w566, y=w567) -> (x*y=→"Dp_d (Mavg)":fxp<+/-,36,14>)
  }
  n332 = while "Quadrature drive_p" {
    stop <- FALSE stop-if-true
    n333 = local read "omega_p (rad/s)"() -> (w627:fxp<+/-,36,13>)
    n334 = local read "Fp_PID"() -> (w623:fxp<+/-,36,16>)
    n335 = call "Oriental_step_motor_PKP225.vi"("F_Threshold"=fxp<+,12,12> 10.0, "dFmr"=fxp<+/-,25,15> 0.0, "omega"=w627, "Fmr"=w623) -> ("vq_F"=→"vq_p_F":fxp<+/-,20,5>, "vd_F"=→"vd_p_F":fxp<+/-,20,5>)  [unwired: 6 in]
  }
  n336 = while "PID force controller_p" {
    shift-right: [w638] -> _
    shift-left: _ -> [w637]
    stop <- FALSE stop-if-true
    n337 = local read "D_p(mm)"() -> (w632:fxp<+/-,32,7>)
    n338 = local read "Dpr_for"() -> (w633:fxp<+/-,22,7>)
    n339 = call "Tick Count7"() -> ("Tick Count(uSec)"=w638:u32)
    n340 = Subtract(x=w638, y=w637) -> (x-y=w636:u32)
    n341 = Subtract(x=w633, y=w632) -> (x-y=w631:fxp<+/-,33,8>)
    n342 = Multiply(x="Kp_p", y=w631) -> (x*y=→"Fp_PID":fxp<+/-,64,20>)
    n343 = Divide(x=u32 1000, y=w636) -> (x/y=→"PID (kHz)":fxp<+/-,20,7>)
  }
  n344 = while "All switch" {
    stop <- FALSE stop-if-true
    n345 = case shown="True" "Encoder reset" {
      frame False {
        n346 = local write "Encoder reset_p"(FALSE ("Encoder reset_p")) -> ()
        n347 = local write "Encoder reset_y"(FALSE ("Encoder reset_y")) -> ()
      }
      frame True {
        n348 = flat-sequence {
          frame #0 {
            n349 = local write "Encoder reset_p"(TRUE ("Encoder reset_p")) -> ()
          }
          frame #1 {
            n350 = local write "Encoder reset_y"(TRUE ("Encoder reset_y")) -> ()
            n351 = local write "Encoder reset_p"(FALSE ("Encoder reset_p")) -> ()
          }
          frame #2 {
            n352 = local write "Encoder reset_y"(FALSE ("Encoder reset_y")) -> ()
          }
        }
      }
    }
  }
  n353 = while "Encoder_y" {
    shift-right: [w685] -> _
    shift-left: _ -> [w677]
    shift-right: [w684] -> _
    shift-left: _ -> [w676]
    shift-right: [w675] -> _
    shift-left: _ -> [w673]
    shift-right: [w681] -> _
    shift-left: _ -> [w678]
    shift-right: [w680] -> _
    shift-left: _ -> [w679]
    shift-right: [w674] -> _
    shift-left: _ -> [w672]
    stop <- FALSE stop-if-true
    w662 = fxp<+/-,16,1> 0.0244140625  # 2*50/4096
    w667 = fxp<+/-,20,-5> 0.00048828125  # L/4096
    w670 = fxp<+/-,20,-5> 0.002499997615814209  # L/800
    w652 = fxp<+/-,16,1> 0.125  # 2*50/800
    n354 = xnode "FPGA I/O Node"() -> ("Mod7/DIO2"=w686:bool, "Mod7/DIO3"=w687:bool)  [unwired: 2 in, 2 out]
    n355 = xnode "FPGA I/O Node"() -> ("Mod7/DIO6"=w683:bool, "Mod7/DIO7"=w682:bool)  [unwired: 2 in, 2 out]
    n356 = local read "Encoder reset_y"() -> (w657:bool)
    n357 = call "encoder_sub.vi"("A_pre"=w677, "B_pre"=w676, "Encoder Position_pre"=w673, "A input"=w686, "Encoder Position Reset"="Encoder reset_y", "B input"=w687) -> ("A"=w685:bool, "B"=w684:bool, "Encoder Position (Counts)"=w675:i32)  [unwired: 19 in]
    "Encoder Position_y1" <- w675
    n358 = call "encoder_sub.vi"("A_pre"=w678, "B_pre"=w679, "Encoder Position_pre"=w672, "A input"=w683, "Encoder Position Reset"=w657, "B input"=w682) -> ("A"=w681:bool, "B"=w680:bool, "Encoder Position (Counts)"=w674:i32)  [unwired: 19 in]
    "Encoder Position_y2" <- w674
    n359 = local read "Belt_in_y"() -> (w665:fxp<+/-,6,6>)
    n360 = local read "Belt_in_y"() -> (w669:fxp<+/-,6,6>)
    n361 = local read "Belt_out_y"() -> (w663:fxp<+/-,7,7>)
    n362 = Divide(x=w667, y="Mag. factor_y") -> (x/y=w666:fxp<+/-,41,13>)
    n363 = local read "Belt_out_y"() -> (w668:fxp<+/-,7,7>)
    n364 = To Fixed-Point(number=w674) -> (fixed-point=w649:fxp<+/-,32,32>)  [unwired: 1 in]
    n365 = local read "Mag. factor_y"() -> (w661:fxp<+/-,20,3>)
    n366 = To Fixed-Point(number=w675) -> (fixed-point=w653:fxp<+/-,32,32>)  [unwired: 1 in]
    n367 = Multiply(x=w666, y=w665) -> (x*y=w664:fxp<+/-,46,18>)
    n368 = Multiply(x=w670, y=w669) -> (x*y=w671:fxp<+/-,26,1>)
    n369 = Divide(x=w664, y=w663) -> (x/y=w651:fxp<+/-,53,18>)
    n370 = Divide(x=w671, y=w668) -> (x/y=w655:fxp<+/-,33,1>)
    n371 = Divide(x=w662, y=w661) -> (x/y=w648:fxp<+/-,32,1>)
    n372 = Multiply(x=w651, y=w649) -> (x*y=→"D_y2":fxp<+/-,37,7>)
    n373 = Multiply(x=w653, y=w652) -> (x*y=→"rad_y1":fxp<+/-,33,20>)
    n374 = Multiply(x=w655, y=w653) -> (x*y=→"D_y1":fxp<+/-,32,7>)
    n375 = Multiply(x=w649, y=w648) -> (x*y=→"rad_y2":fxp<+/-,33,20>)
  }
  n376 = while "Omega_y(T method)" {
    shift-right: [w714] -> _
    shift-left: _ -> [w715]
    shift-right: [w691] -> _
    shift-left: _ -> [w717]
    shift-right: [w719] -> _
    shift-left: _ -> [w720]
    shift-right: [w707] -> _
    shift-left: _ -> [w705]
    shift-right: [w700] -> _
    shift-left: _ -> [w706]
    shift-right: [w703] -> _
    shift-left: _ -> [w704]
    stop <- FALSE stop-if-true
    w698 = fxp<+/-,32,0> 0.3183098859153688  # L/2/pi
    w709 = fxp<+,32,0> 0.1953125  # 800/4096
    w713 = fxp<+/-,32,0> 0.3183098859153688  # L/2/pi
    n377 = local read "Encoder Position_y1"() -> (w714:i32)
    n378 = call "Tick Count2"() -> ("Tick Count(Ticks)"=w701:u32)
    n379 = local read "Encoder Position_y2"() -> (w707:i32)
    n380 = local read "Mag. factor_y"() -> (w708:fxp<+/-,20,3>)
    n381 = call "omega_sub_Encoder_800ppr.vi"("mt0"="mt0_omega_y", "omega_pre"=w717, "ticks_m_pre"=w720, "ticks"=w701, "count_pre"=w715, "count"=w714) -> ("ticks_m"=w719:u32, "mt"=→"mt_omega_y1":u32, "omega"=w691:fxp<+/-,36,13>)  [unwired: 3 in]
    "omega_y1 (T)" <- w691
    n382 = call "omega_sub_Encoder_800ppr.vi"("omega_pre"=w706, "ticks_m_pre"=w704, "ticks"=w701, "count_pre"=w705, "count"=w707) -> ("ticks_m"=w703:u32, "mt"=→"mt_omega_y2":u32, "omega"=w700:fxp<+/-,36,13>)  [unwired: 4 in]
    n383 = local read "Belt_in_y"() -> (w697:fxp<+/-,6,6>)
    n384 = local read "Belt_out_y"() -> (w695:fxp<+/-,7,7>)
    n385 = Divide(x=w709, y=w708) -> (x/y=w699:fxp<+/-,32,1>)
    n386 = Multiply(x=w713, y="Belt_in_y") -> (x*y=w711:fxp<+/-,38,6>)
    n387 = Multiply(x=w698, y=w697) -> (x*y=w696:fxp<+/-,38,6>)
    n388 = Divide(x=w696, y=w695) -> (x/y=w689:fxp<+/-,45,6>)
    n389 = Divide(x=w711, y="Belt_out_y") -> (x/y=w692:fxp<+/-,20,1>)
    n390 = Multiply(x=w700, y=w699) -> (x*y=w688:fxp<+/-,36,13>)
    "omega_y2 (T)" <- w688
    n391 = Multiply(x=w692, y=w691) -> (x*y=→"Dy1_d (T)":fxp<+/-,36,13>)
    n392 = Multiply(x=w689, y=w688) -> (x*y=→"Dy2_d (T)":fxp<+/-,36,13>)
  }
  n393 = while {
    stop <- FALSE stop-if-true
    n394 = case shown="True" "Set 3" {
      frame False {
      }
      frame True {
        n395 = local write "Kp_p"(fxp<+/-,36,9> 100.0 ("Kp_p")) -> ()
        n396 = local write item#-1(fxp<+,22,6> 3.0 ("fp_tolorance")) -> ()
      }
    }
    n397 = case shown="True" "Set 2" {
      frame False {
      }
      frame True {
        n398 = local write "Kp_p"(fxp<+/-,36,9> 50.0 ("Kp_p")) -> ()
        n399 = local write item#-1(fxp<+,22,6> 1.5 ("fp_tolorance")) -> ()
      }
    }
    n400 = case shown="True" "Set 1" {
      frame False {
      }
      frame True {
        n401 = local write "Kp_p"(fxp<+/-,36,9> 50.0 ("Kp_p")) -> ()
        n402 = local write item#-1(fxp<+,22,6> 3.0 ("fp_tolorance")) -> ()
      }
    }
    n403 = case shown="True" "Set 5" {
      frame False {
      }
      frame True {
        n404 = local write "Kp_p"(fxp<+/-,36,9> 150.0 ("Kp_p")) -> ()
        n405 = local write item#-1(fxp<+,22,6> 3.0 ("fp_tolorance")) -> ()
      }
    }
    n406 = case shown="True" "Set 6" {
      frame False {
      }
      frame True {
        n407 = local write "Kp_p"(fxp<+/-,36,9> 150.0 ("Kp_p")) -> ()
        n408 = local write item#-1(fxp<+,22,6> 1.5 ("fp_tolorance")) -> ()
      }
    }
    n409 = case shown="True" "Set 4" {
      frame False {
      }
      frame True {
        n410 = local write "Kp_p"(fxp<+/-,36,9> 100.0 ("Kp_p")) -> ()
        n411 = local write item#-1(fxp<+,22,6> 1.5 ("fp_tolorance")) -> ()
      }
    }
  }
  n412 = while {
    stop <- FALSE stop-if-true
    n413 = local read "omega_p (Mavg)"() -> (w743:fxp<+/-,36,14>)
    n414 = xnode "Butterworth Filter"("input data"=w743, "scaled coefficients"="scaled coefficients") -> ("output data"=→"omega_p (Mavg w. f)":fxp<+/-,36,18>)  [unwired: 1 in]
  }
